vi "TextCommand.vi"() -> ()   [LabVIEW 2012]
panel:
  out "element":string
  in  "string":string="*IDN?"
  out "Bytes at Serial Port":u32
  out "error out":errorcluster
  out "return count":u32
  out "VISA resource name out":refnum<visa-resource-name>
  out "read buffer":string
  in  "byte count":u32=99
  in  "VISA resource name":refnum<visa-resource-name>
  # ":syst:err?"
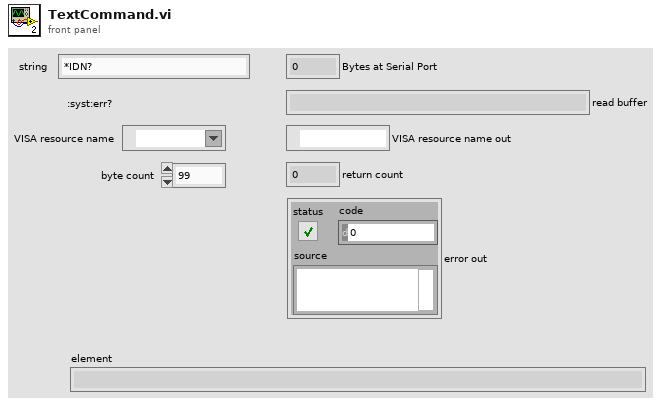
[diagram p1: front panel]
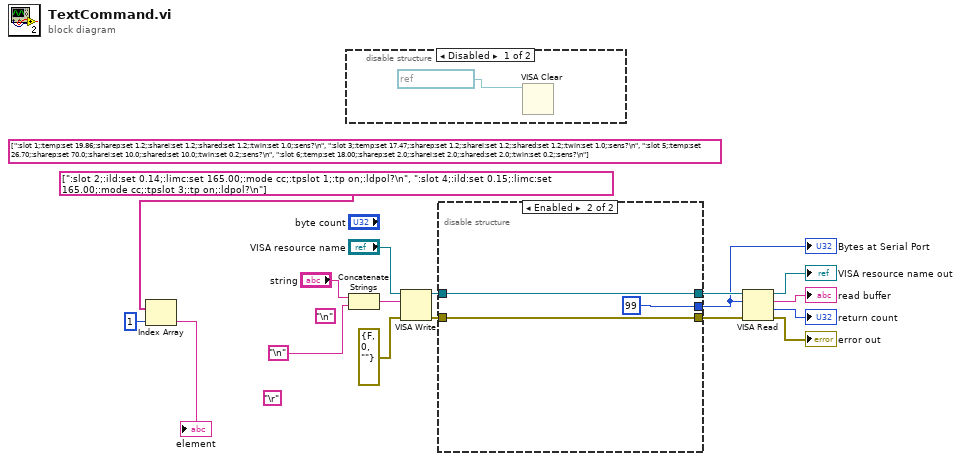
[diagram p0: block diagram]
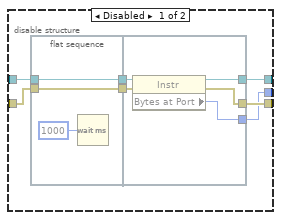
[diagram p2: hidden frame]
diagram:
  (unwired) string[] [":slot 1;:temp:set 19.86;:sharep:set 1.2;:sharei:set 1.2;:shared:set 1.2;:twin:set 1.0;:sens?\n", ":slot 3;:temp:set 17.47;:sharep:set 1.2;:sharei:set 1.2;:shared:set 1.2;:twin:set 1.0;:sens?\n", ":slot 5;:temp:set 26.70;:sharep:set 70.0;:sharei:set 10.0;:shared:set 10.0;:twin:set 0.2;:sens?\n", ":slot 6;:temp:set 18.00;:sharep:set 2.0;:sharei:set 2.0;:shared:set 2.0;:twin:set 0.2;:sens?\n"] ("TEC Strings")
  (unwired) "\r"
  (unwired) "\n"
  n1 = Index Array(array=string[] [":slot 2;:ild:set 0.14;:limc:set 165.00;:mode cc;:tpslot 1;:tp on;:ldpol?\n", ":slot 4;:ild:set 0.15;:limc:set 165.00;:mode cc;:tpslot 3;:tp on;:ldpol?\n"] ("LD Strings"), index=1) -> (element=→"element":string)
  n2 = disable-structure shown="Disabled" {
    frame Disabled {
      n3 = VISA Clear(VISA resource name=refnum<visa-resource-name> "ThorLabs" ("VISA resource name 2")) -> ()  [unwired: 1 in, 2 out]
    }
    frame Enabled {
    }
  }
  n4 = Concatenate Strings("string", "\n") -> (w14:string)
  n5 = VISA Write(VISA resource name="VISA resource name", write buffer=w14, error in (no error)=errorcluster {"status"=FALSE, "code"=0, "source"=""}) -> (VISA resource name out=w10:refnum<visa-resource-name>, error out=w8:errorcluster)  [unwired: 1 out]
  n6 = disable-structure shown="Enabled" {
    disable-tunnel: w10 -> [w23 w36]
    disable-tunnel: [w22 w36] -> w9
    disable-tunnel: w8 -> [w21 w35]
    disable-tunnel: [w20 w35] -> w7
    disable-tunnel: [w19 u32 99 ("Bytes at Serial Port")] -> w6
    frame Disabled {
      n7 = flat-sequence {
        tunnel: w21 -> [w27]
        tunnel: w23 -> [w28]
        tunnel: [w28] -> w25
        tunnel: [w27] -> w24
        tunnel: [w32] -> w22
        tunnel: [w30] -> w20
        tunnel: [w29] -> w19
        tunnel: w25 -> [w33]
        tunnel: w24 -> [w31]
        frame #0 {
          n8 = Wait (ms)(milliseconds to wait=u32 1000) -> ()  [unwired: 1 out]
        }
        frame #1 {
          n9 = property class="Instr"(reference=w33, error in=w31) -> (reference out=w32:refnum<visa-resource-name>, error out=w30:errorcluster, "Bytes at Port"=w29:u32)
        }
      }
    }
    frame Enabled {
    }
  }
  "Bytes at Serial Port" <- w6
  n10 = VISA Read(VISA resource name=w9, byte count=w6, error in (no error)=w7) -> (VISA resource name out=→"VISA resource name out":refnum<visa-resource-name>, read buffer=→"read buffer":string, return count=→"return count":u32, error out=→"error out":errorcluster)
